vi "Define Mode Release Event.vi"(8 "error in (no error)":errorcluster, 11 "user event in":refnum<user-event>) -> (0 "error out":errorcluster, 2 "function return":i32)   [LabVIEW 2014, in "Interrupt.lvlib"]
doc: "int Define_Mode_Release_Event(void *eventRef);"
uses:
  Interrupt.lvlib
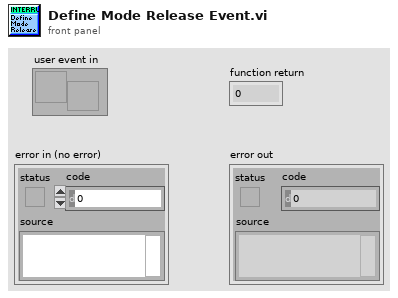
[diagram p1: front panel]
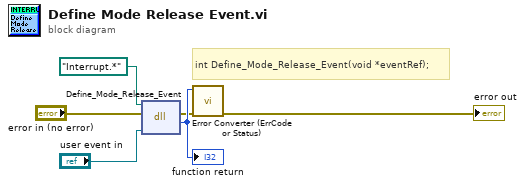
[diagram p0: block diagram]
diagram:
  # "int Define_Mode_Release_Event(void *eventRef);"
  n1 = dll-call lib="C:/Users/ktalke/Documents/RC-Jessie-Examples/Interrupt/Interrupt.so" fn="Define_Mode_Release_Event"(path in=path "Interrupt.*", error in="error in (no error)", "eventRef"="user event in") -> (error out=w4:errorcluster, "return type"=w6:i32)  [unwired: 2 in, 1 out]
  "function return" <- w6
  n2 = call "Error Converter (ErrCode or Status).vi"("error in (no error)"=w4, "error code"=w6) -> ("error out"=→"error out":errorcluster)  [unwired: 9 in]
